vi "spi_full_control.vi"(0 "connection ID":refnum<k5>, 1 "Device":u16(ring) items=["Attenuation", "Clipping", "Enable channel", "Delay line", "ASIC", "Enable L1 ch", "ASIC L1"], 2 "Read/#write":bool, 3 "Data":i32=72, 4 "Register or channel":i32=72, 5 "error out 3":errorcluster, 6 "Read physical":bool, 7 "Id in":i32, 8 "chip delay":i32) -> (9 "Data to send hex":string, 11 "Data to send dec":u32, 13 "hex integer string":string, 14 "connection ID out":refnum<k5>, 15 "Id out":i32=72, 16 "data out serial":string, 17 "data read value":u32, 19 "error out 2":errorcluster)   [LabVIEW 2012]
panel:
  out "Data out 2":string
  out "Data out":string
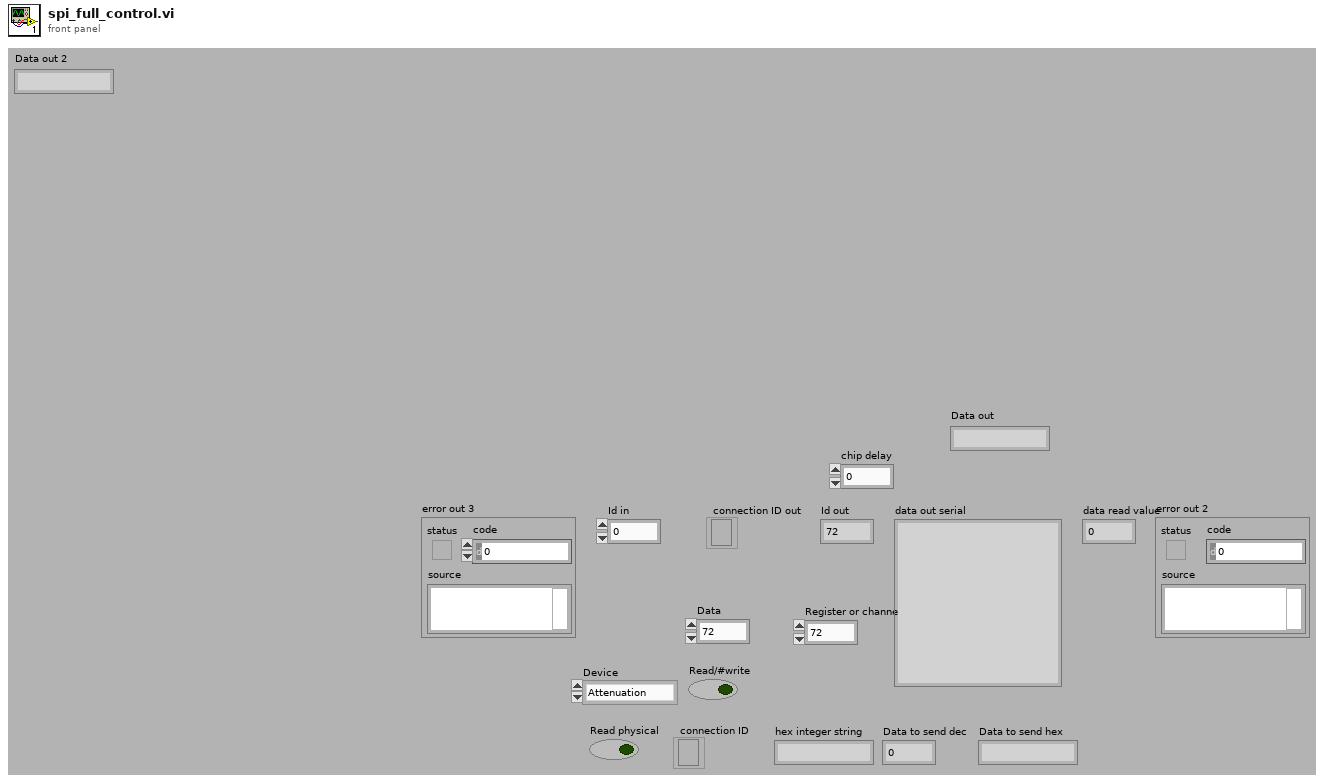
[diagram p1: front panel]
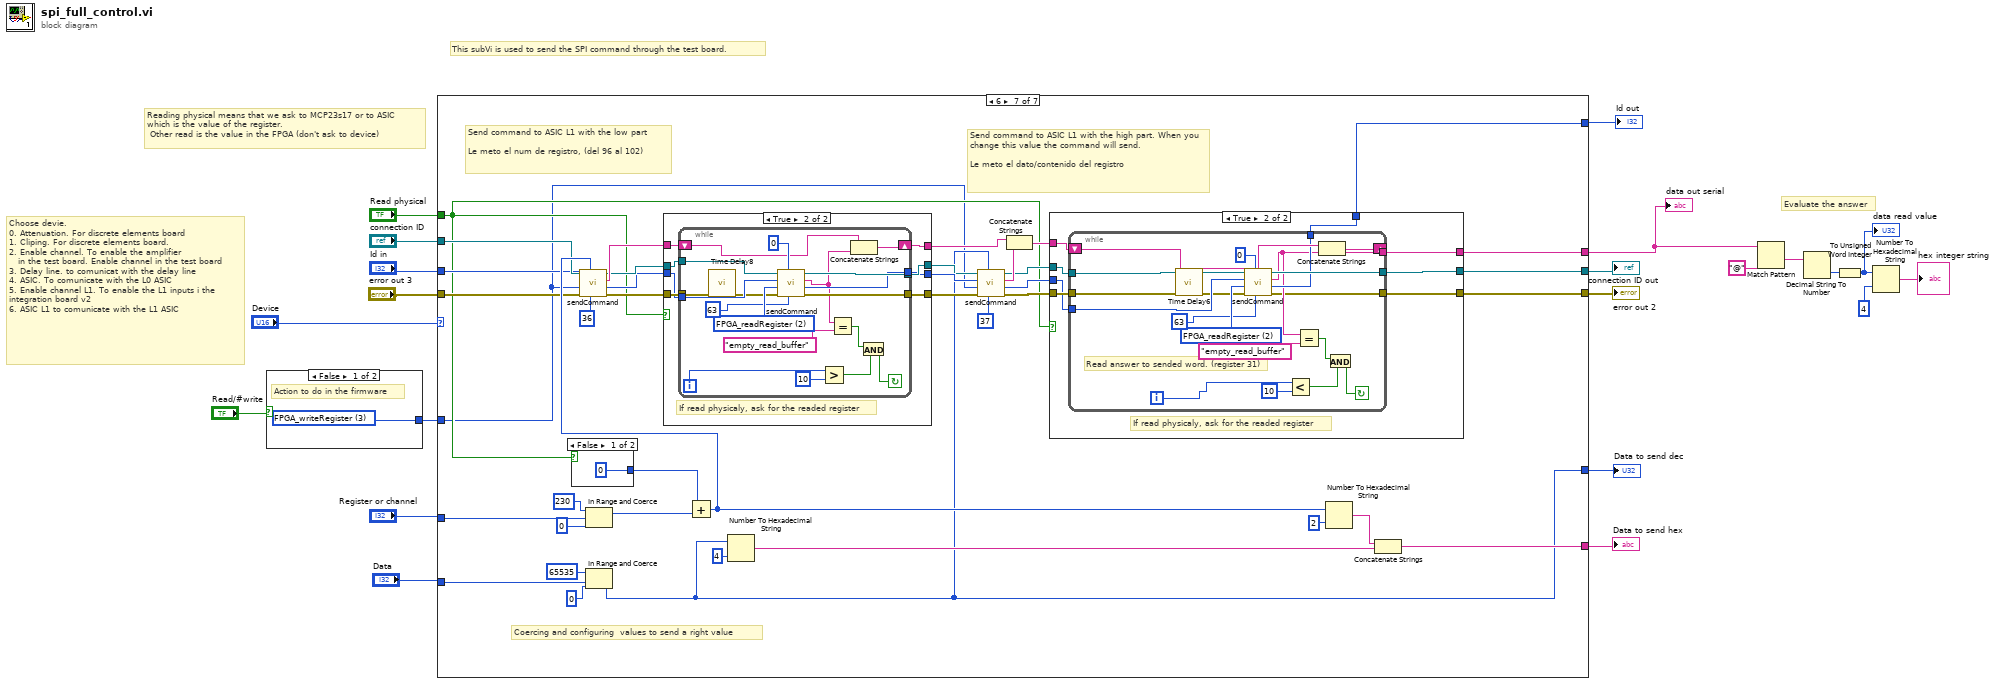
[diagram p0: block diagram]
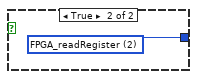
[diagram p2: hidden frame]
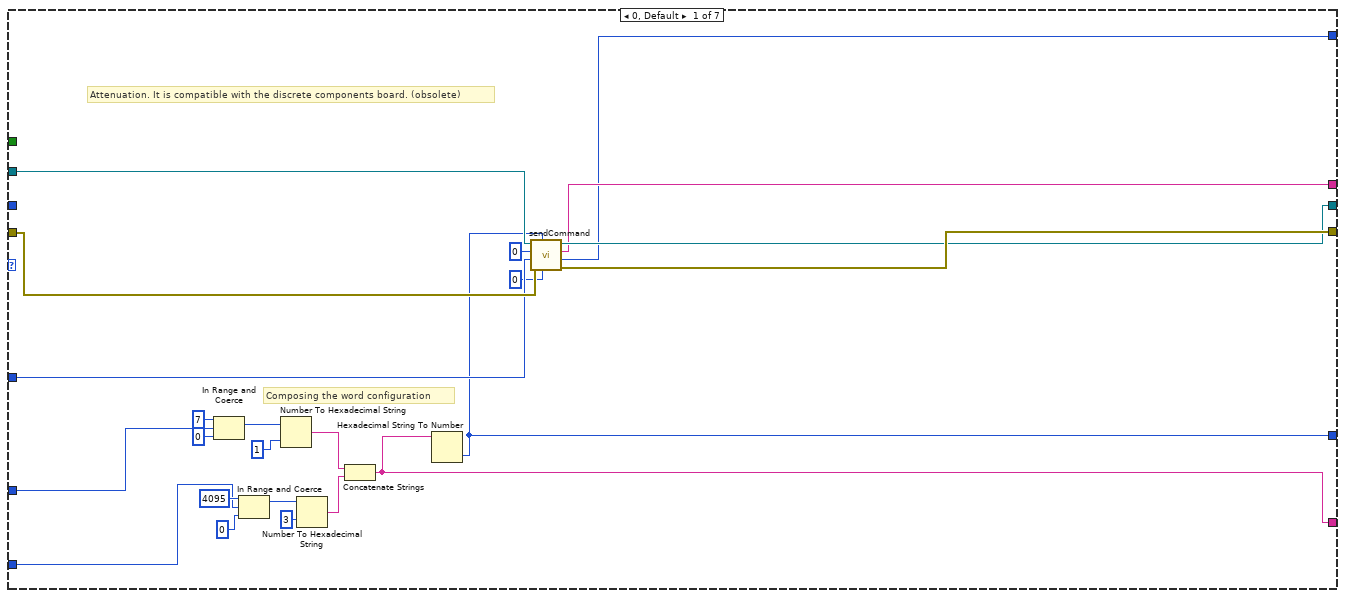
[diagram p3: hidden frame]
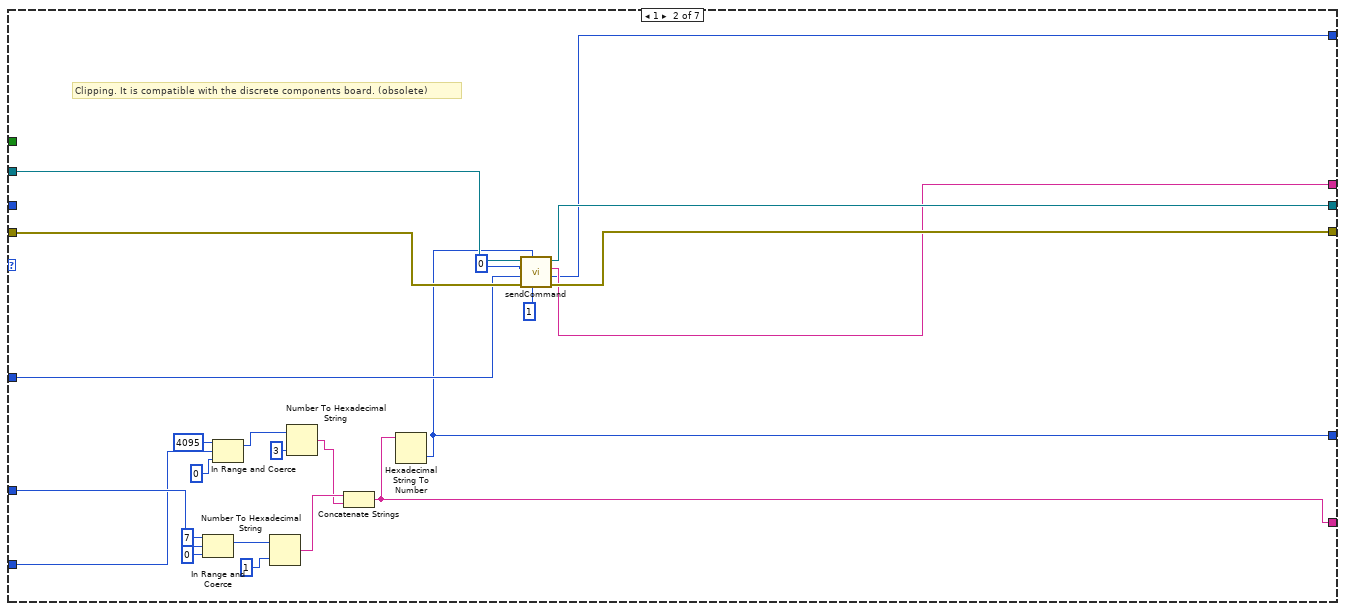
[diagram p4: hidden frame]
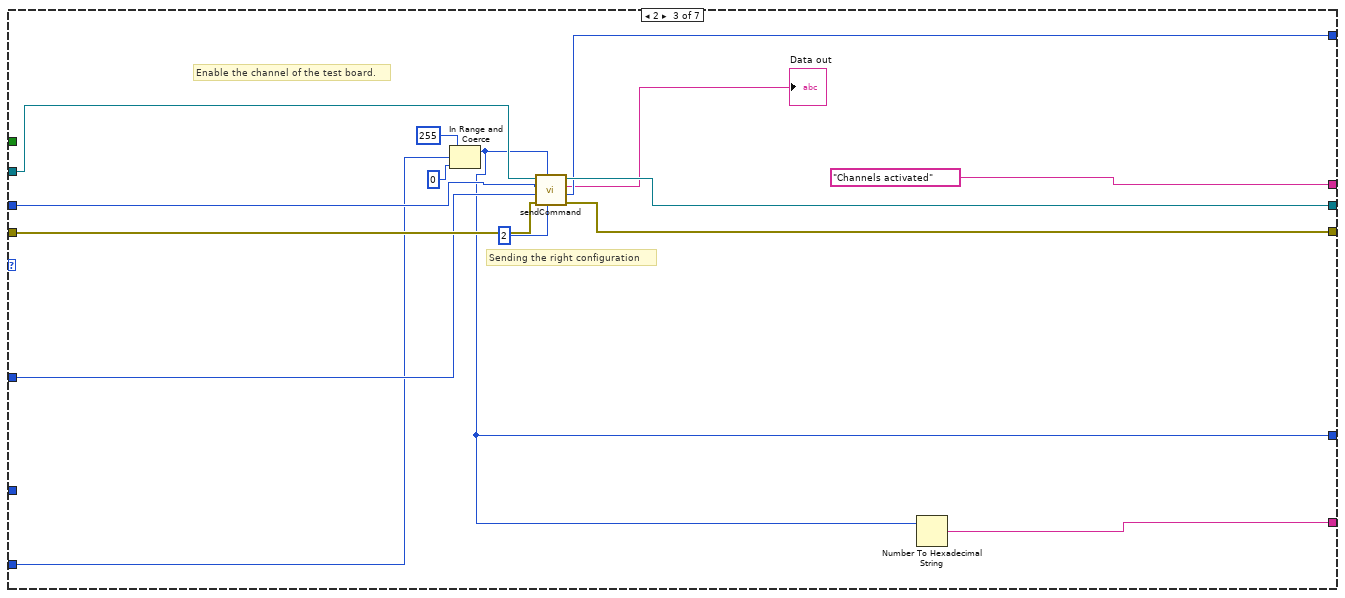
[diagram p5: hidden frame]
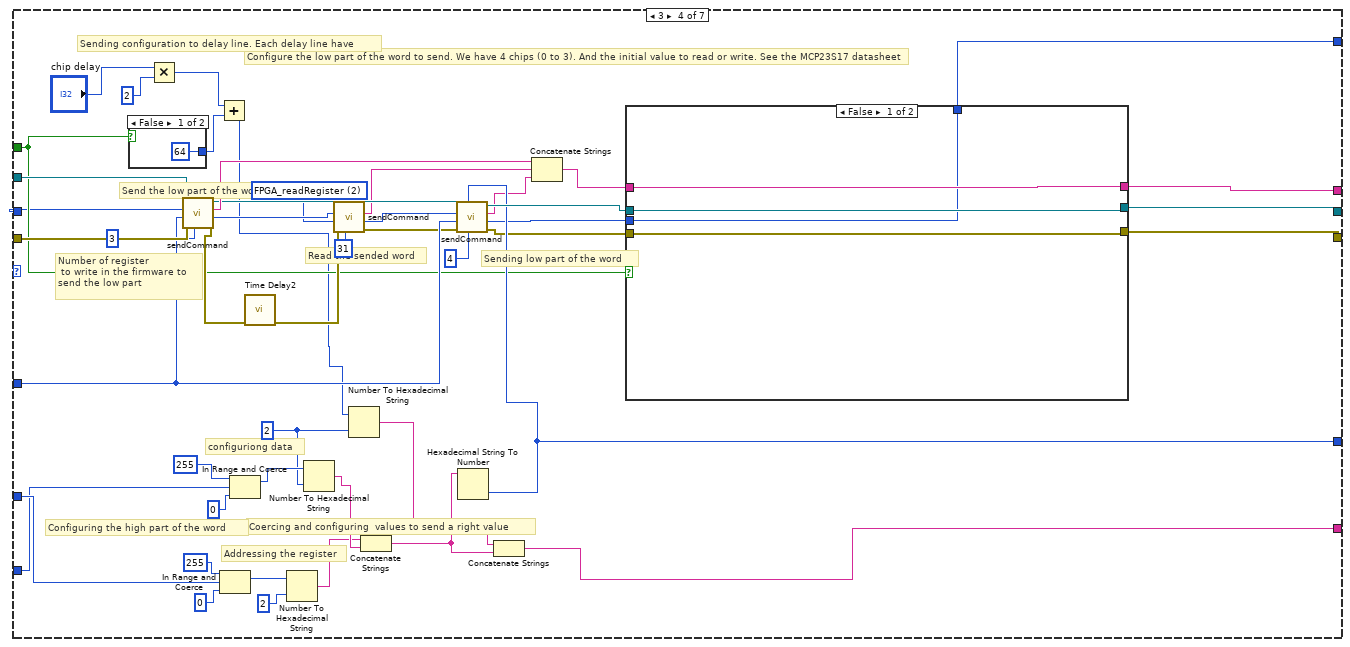
[diagram p6: hidden frame]
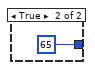
[diagram p7: hidden frame]
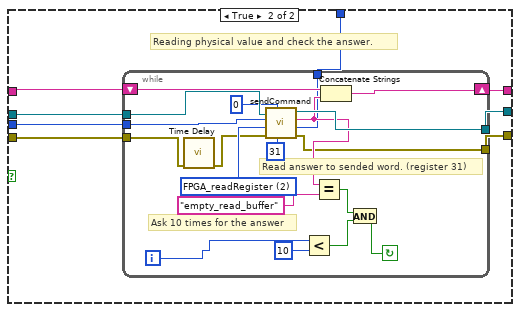
[diagram p8: hidden frame]
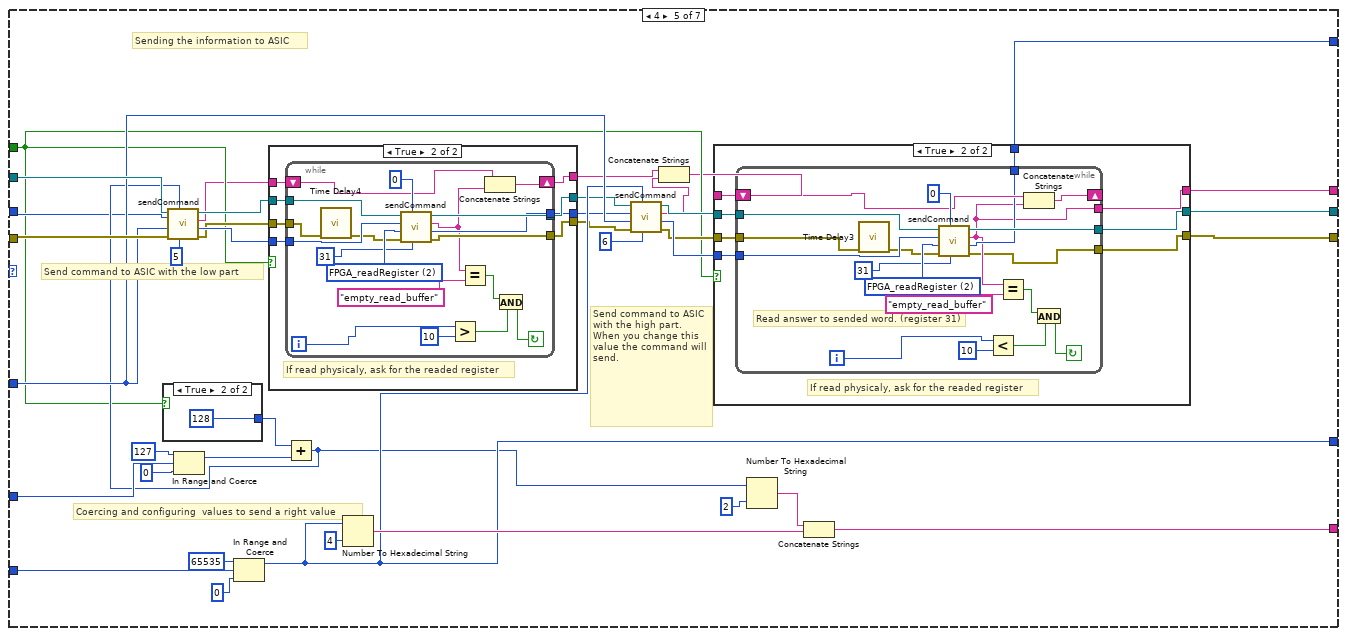
[diagram p9: hidden frame]
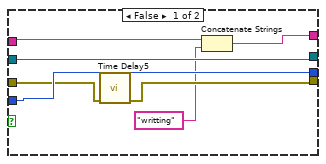
[diagram p10: hidden frame]
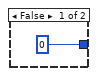
[diagram p11: hidden frame]
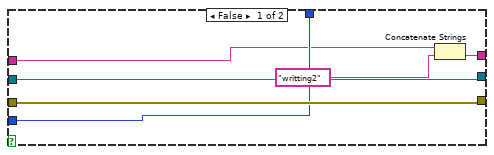
[diagram p12: hidden frame]
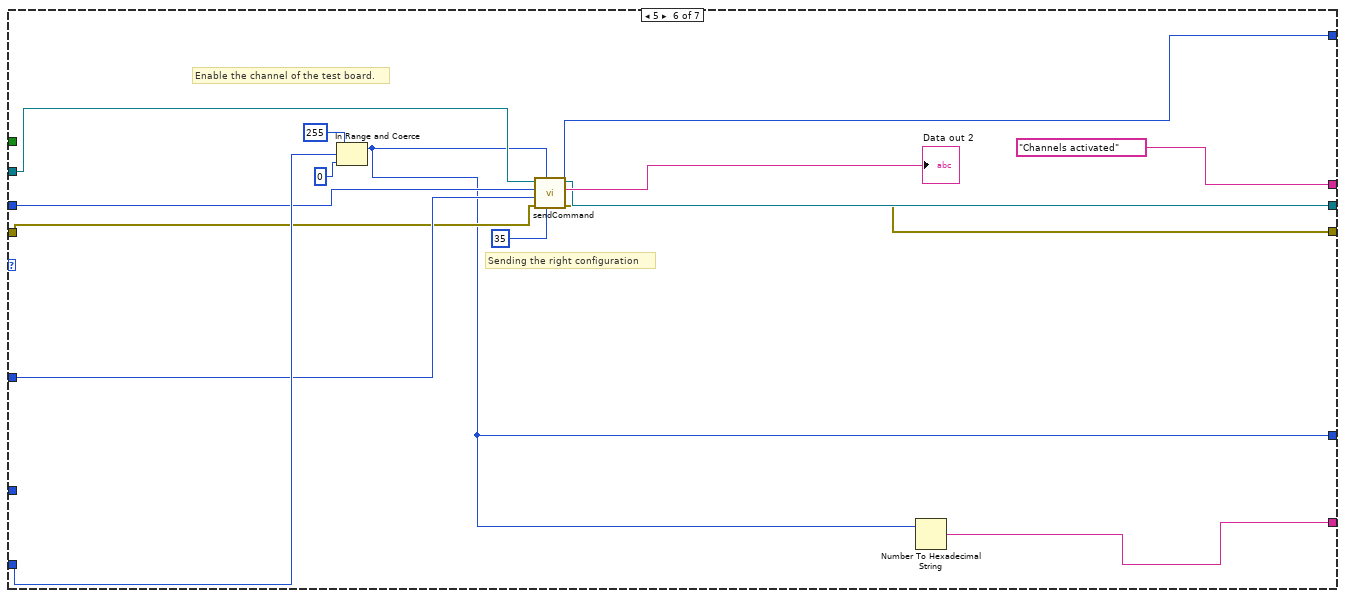
[diagram p13: hidden frame]
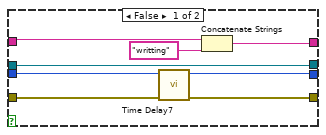
[diagram p14: hidden frame]
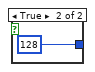
[diagram p15: hidden frame]
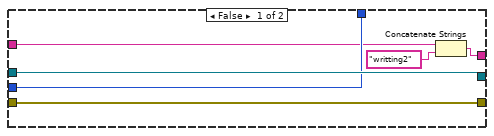
[diagram p16: hidden frame]
diagram:
  # "Reading physical means that we ask to MCP23s17 or to ASIC \nwhich is the value of the register.\n Other read is the value in the FPGA (don't ask to device)"
  # "Evaluate the answer"
  # "Choose devie.\n0. Attenuation. For discrete elements board\n1. Cliping. For discrete elements board.\n2. Enable channel. To enable the amplifier \n   in the test board. Enable channel in the test board\n3. Delay line. to comunicat with the delay line\n4. ASIC. To comunicate with the L0 ASIC\n5. Enable channel L1. To enable the L1 inputs i the integration board v2\n6. ASIC L1 to comunicate with the L1 ASIC"
  # "This subVi is used to send the SPI command through the test board."
  n1 = case shown="False" "Read/#write" {
    tunnel: [w22 w23] -> w9
    frame False {
      w22 = u16 3 items=["sendCommand"=9, "FPGA_writeRegister"=3, "FPGA_readRegister"=2, "uC_writeRegister"=1, "uC_readRegister"=0] ("Action")
      # "Action to do in the firmware"
    }
    frame True {
      w23 = u16 2 items=["sendCommand"=9, "FPGA_writeRegister"=3, "FPGA_readRegister"=2, "uC_writeRegister"=1, "uC_readRegister"=0] ("Action")
    }
  }
  n2 = case shown="6" "Device" {
    tunnel: [w44 w67 w80 w106 w179 w276 w298] -> w7
    tunnel: "error out 3" -> [w45 w69 w83 w132 w192 w282 w292]
    tunnel: "connection ID" -> [w46 w68 w82 w131 w193 w280 w294]
    tunnel: [w43 w66 w81 w105 w187 w277 w297] -> w6
    tunnel: w9 -> [w31 w63 w79 w130 w191 w283 w289]
    tunnel: "Register or channel" -> [w26 w62 _ w118 w189 _ w301]
    tunnel: "Data" -> [w27 w57 w75 w117 w190 w284 w300]
    tunnel: [w25 w48 "Channels activated" ("data out") w104 w180 "Channels activated" ("data out") w296] -> w18
    tunnel: [w29 w50 w74 w116 w184 w279 w291] -> w13
    tunnel: [w28 w49 w72 w111 w188 w278 w299] -> w14
    tunnel: "Read physical" -> [_ _ _ w91 w172 _ w290]
    tunnel: "Id in" -> [_ _ w78 w85 w182 w281 w293]
    tunnel: [w24 w47 w71 w92 w170 w274 w295] -> w3
    frame 0, Default {
      # "Attenuation. It is compatible with the discrete components board. (obsolete)"
      # "Composing the word configuration"
      n3 = In Range and Coerce(upper limit=7, x=w26, lower limit=0) -> (coerced(x)=w41:i32)  [unwired: 1 out]
      n4 = In Range and Coerce(upper limit=4095, x=w27, lower limit=0) -> (coerced(x)=w37:i32)  [unwired: 1 out]
      n5 = Number To Hexadecimal String(1:i16 1 ("width (-)"), 2:w41) -> (0:w34:string)
      n6 = Number To Hexadecimal String(1:i16 3 ("width (-)"), 2:w37) -> (0:w33:string)
      n7 = Concatenate Strings(w34, w33) -> (w28:string)
      n8 = Hexadecimal String To Number(string=w28) -> (number=w29:u32)  [unwired: 2 in, 1 out]
      n9 = call "sendCommand.vi"("Address"=0, "Data"=w29, "error in"=w45, "Action"=w31, "id_in"=0, "connection ID"=w46) -> ("error out"=w44:errorcluster, "id_out"=w24:i32, "Data out"=w25:string, "connection ID out"=w43:refnum<k5>)  [unwired: 1 in, 1 out]
    }
    frame 1 {
      # "Clipping. It is compatible with the discrete components board. (obsolete)"
      n10 = In Range and Coerce(upper limit=7, x=w62, lower limit=0) -> (coerced(x)=w61:i32)  [unwired: 1 out]
      n11 = In Range and Coerce(upper limit=4095, x=w57, lower limit=0) -> (coerced(x)=w56:i32)  [unwired: 1 out]
      n12 = Number To Hexadecimal String(1:i16 1 ("width (-)"), 2:w61) -> (0:w53:string)
      n13 = Number To Hexadecimal String(1:i16 3 ("width (-)"), 2:w56) -> (0:w52:string)
      n14 = Concatenate Strings(w53, w52) -> (w49:string)
      n15 = Hexadecimal String To Number(string=w49) -> (number=w50:u32)  [unwired: 2 in, 1 out]
      n16 = call "sendCommand.vi"("Address"=1, "Data"=w50, "error in"=w69, "Action"=w63, "id_in"=0 ("id"), "connection ID"=w68) -> ("error out"=w67:errorcluster, "id_out"=w47:i32, "Data out"=w48:string, "connection ID out"=w66:refnum<k5>)  [unwired: 1 in, 1 out]
    }
    frame 2 {
      # "Sending the right configuration"
      # "Enable the channel of the test board."
      n17 = In Range and Coerce(upper limit=255, x=w75, lower limit=0) -> (coerced(x)=w74:i32)  [unwired: 1 out]
      n18 = call "sendCommand.vi"("Address"=2, "Data"=w74, "error in"=w83, "Action"=w79, "id_in"=w78, "connection ID"=w82) -> ("error out"=w80:errorcluster, "id_out"=w71:i32, "Data out"=→"Data out":string, "connection ID out"=w81:refnum<k5>)  [unwired: 1 in, 1 out]
      n19 = Number To Hexadecimal String(2:w74) -> (0:w72:string)  [unwired: 1 in]
    }
    frame 3 {
      w97 = u16 2 items=["sendCommand"=9, "FPGA_writeRegister"=3, "FPGA_readRegister"=2, "uC_writeRegister"=1, "uC_readRegister"=0] ("Action")
      w114 = i16 2 ("width (-)")
      # "Coercing and configuring  values to send a right value"
      # "Number of register\n to write in the firmware to \nsend the low part"
      # "Sending low part of the word"
      # "configuriong data"
      # "Addressing the register"
      # "Configuring the high part of the word"
      # "Read the sended word"
      # "Send the low part of the word"
      # "Configure the low part of the word to send. We have 4 chips (0 to 3). And the initial value to read or write. See the MCP23S17 datasheet"
      # "Sending configuration to delay line. Each delay line have"
      n20 = case shown="False" w91 {
        tunnel: [64 ("Address") 65 ("Address")] -> w88
        frame False {
        }
        frame True {
        }
      }
      n21 = Multiply(x="chip delay", y=2) -> (x*y=w89:i32)
      n22 = Add(x=w89, y=w88) -> (x+y=w87:i32)
      n23 = call "sendCommand.vi"("Address"=3, "Data"=w87, "error in"=w132, "Action"=w130, "id_in"=w85, "connection ID"=w131) -> ("error out"=w93:errorcluster, "id_out"=w100:i32, "Data out"=w110:string, "connection ID out"=w102:refnum<k5>)  [unwired: 1 in, 1 out]
      n24 = In Range and Coerce(upper limit=255, x=w118, lower limit=0) -> (coerced(x)=w126:i32)  [unwired: 1 out]
      n25 = In Range and Coerce(upper limit=255, x=w117, lower limit=0) -> (coerced(x)=w122:i32)  [unwired: 1 out]
      n26 = call "Time Delay2"("error in (no error)"=w93) -> ("error out"=w94:errorcluster)  [unwired: 10 in]
      n27 = Number To Hexadecimal String(1:i16 2 ("width (-)"), 2:w126) -> (0:w115:string)
      n28 = Number To Hexadecimal String(1:w114, 2:w122) -> (0:w119:string)
      n29 = call "sendCommand.vi"("Address"=31, "error in"=w94, "Action"=w97, "id_in"=w100, "connection ID"=w102) -> ("error out"=w103:errorcluster, "id_out"=w99:i32, "Data out"=w98:string, "connection ID out"=w101:refnum<k5>)  [unwired: 2 in, 1 out]
      n30 = Number To Hexadecimal String(1:w114, 2:w87) -> (0:w113:string)
      n31 = Concatenate Strings(w115, w119) -> (w112:string)
      n32 = Hexadecimal String To Number(string=w112) -> (number=w116:u32)  [unwired: 2 in, 1 out]
      n33 = call "sendCommand.vi"("Address"=4, "Data"=w116, "error in"=w103, "Action"=w130, "id_in"=w99, "connection ID"=w101) -> ("error out"=w95:errorcluster, "id_out"=w107:i32, "Data out"=w109:string, "connection ID out"=w127:refnum<k5>)  [unwired: 1 in, 1 out]
      n34 = Concatenate Strings(w113, w112) -> (w111:string)
      n35 = Concatenate Strings(w110, w98, w109) -> (w108:string)
      n36 = case shown="False" w91 {
        tunnel: w127 -> [w137 w146]
        tunnel: w95 -> [w138 w145]
        tunnel: [w138 w142] -> w106
        tunnel: [w137 w143] -> w105
        tunnel: [w136 w144] -> w104
        tunnel: w108 -> [w136 w141]
        tunnel: w107 -> [w135 w140]
        tunnel: [w135 w139] -> w92
        frame False {
        }
        frame True {
          # "Reading physical value and check the answer."
          n37 = while {
            tunnel: w145 -> [w149]
            tunnel: [w150] -> w142
            tunnel: [w155] -> w143
            tunnel: w146 -> [w159]
            shift-right: [w152] -> w144
            shift-left: w141 -> [w154]
            tunnel: w140 -> [w151]
            tunnel: [w147] -> w139
            i -> [w160]
            stop <- w161 continue-if-true
            w158 = u16 2 items=["sendCommand"=9, "FPGA_writeRegister"=3, "FPGA_readRegister"=2, "uC_writeRegister"=1, "uC_readRegister"=0] ("Action 2")
            # "Read answer to sended word. (register 31)"
            # "Ask 10 times for the answer"
            n38 = call "Time Delay"("error in (no error)"=w149) -> ("error out"=w148:errorcluster)  [unwired: 10 in]
            n39 = call "sendCommand.vi"("Address"=31, "Data"=0, "error in"=w148, "Action"=w158, "id_in"=w151, "connection ID"=w159) -> ("error out"=w150:errorcluster, "id_out"=w147:i32, "Data out"=w153:string, "connection ID out"=w155:refnum<k5>)  [unwired: 1 in, 1 out]
            n40 = Less?(x=w160, y=10) -> (x < y?=w163:bool)
            n41 = Equal?(x=w153, y="empty_read_buffer") -> (x = y?=w164:bool)
            n42 = Concatenate Strings(w154, w153) -> (w152:string)
            n43 = And(x=w164, y=w163) -> (x .and. y?=w161:bool)
          }
        }
      }
    }
    frame 4 {
      # "Coercing and configuring  values to send a right value"
      # "Send command to ASIC with the high part. When you change this value the command will send."
      # "Send command to ASIC with the low part"
      # "Sending the information to ASIC"
      n44 = case shown="True" w172 {
        tunnel: [0 ("Address") 128 ("Address")] -> w186
        frame False {
        }
        frame True {
        }
      }
      n45 = In Range and Coerce(upper limit=127, x=w189, lower limit=0) -> (coerced(x)=w185:i32)  [unwired: 1 out]
      n46 = In Range and Coerce(upper limit=65535, x=w190, lower limit=0) -> (coerced(x)=w184:i32)  [unwired: 1 out]
      n47 = Add(x=w186, y=w185) -> (x+y=w183:i32)
      n48 = call "sendCommand.vi"("Address"=5, "Data"=w183, "error in"=w192, "Action"=w191, "id_in"=w182, "connection ID"=w193) -> ("error out"=w173:errorcluster, "id_out"=w175:i32, "Data out"=w166:string, "connection ID out"=w174:refnum<k5>)  [unwired: 1 in, 1 out]
      n49 = case shown="True" w172 {
        tunnel: w174 -> [w211 w219]
        tunnel: w173 -> [w209 w218]
        tunnel: [w208 w217] -> w177
        tunnel: [w211 w216] -> w176
        tunnel: [w206 w214] -> w169
        tunnel: w175 -> [w210 w215]
        tunnel: [w210 w213] -> w171
        tunnel: w166 -> [w205 w212]
        frame False {
          n50 = call "Time Delay5"("error in (no error)"=w209) -> ("error out"=w208:errorcluster)  [unwired: 10 in]
          n51 = Concatenate Strings(w205, "writting" ("Data out")) -> (w206:string)
        }
        frame True {
          # "If read physicaly, ask for the readed register"
          n52 = while {
            tunnel: w218 -> [w226]
            tunnel: [w224] -> w217
            tunnel: [w232] -> w216
            tunnel: w219 -> [w228]
            tunnel: w215 -> [w231]
            tunnel: [w223] -> w213
            shift-right: [w220] -> w214
            shift-left: w212 -> [w222]
            i -> [w233]
            stop <- w234 continue-if-true
            w230 = u16 2 items=["sendCommand"=9, "FPGA_writeRegister"=3, "FPGA_readRegister"=2, "uC_writeRegister"=1, "uC_readRegister"=0] ("Action 2")
            n53 = call "Time Delay4"("error in (no error)"=w226) -> ("error out"=w225:errorcluster)  [unwired: 10 in]
            n54 = call "sendCommand.vi"("Address"=31, "Data"=0, "error in"=w225, "Action"=w230, "id_in"=w231, "connection ID"=w228) -> ("error out"=w224:errorcluster, "id_out"=w223:i32, "Data out"=w221:string, "connection ID out"=w232:refnum<k5>)  [unwired: 1 in, 1 out]
            n55 = Greater?(x=w233, y=10) -> (0:w236:bool)
            n56 = Equal?(x=w221, y="empty_read_buffer") -> (x = y?=w237:bool)
            n57 = Concatenate Strings(w222, w221) -> (w220:string)
            n58 = And(x=w237, y=w236) -> (x .and. y?=w234:bool)
          }
        }
      }
      n59 = Number To Hexadecimal String(1:i16 4 ("width (-)"), 2:w184) -> (0:w194:string)
      n60 = call "sendCommand.vi"("Address"=6, "Data"=w184, "error in"=w177, "Action"=w191, "id_in"=w171, "connection ID"=w176) -> ("error out"=w178:errorcluster, "id_out"=w181:i32, "Data out"=w168:string, "connection ID out"=w202:refnum<k5>)  [unwired: 1 in, 1 out]
      n61 = Concatenate Strings(w169, w168) -> (w167:string)
      n62 = case shown="True" w172 {
        tunnel: w202 -> [w245 w254]
        tunnel: w178 -> [w246 w253]
        tunnel: [w246 w252] -> w179
        tunnel: [w245 w251] -> w187
        tunnel: [w243 w247] -> w180
        tunnel: w181 -> [w244 w250]
        tunnel: w167 -> [w241 w249]
        tunnel: [w244 w248] -> w170
        frame False {
          n63 = Concatenate Strings(w241, "writting2" ("Data out")) -> (w243:string)
        }
        frame True {
          # "If read physicaly, ask for the readed register"
          n64 = while {
            tunnel: w253 -> [w261]
            tunnel: [w255] -> w252
            tunnel: [w267] -> w251
            tunnel: w254 -> [w263]
            tunnel: w250 -> [w266]
            tunnel: [w257] -> w248
            shift-right: [w259] -> _
            shift-left: w249 -> [w258]
            tunnel: [w256] -> w247
            i -> [w268]
            stop <- w269 continue-if-true
            w265 = u16 2 items=["sendCommand"=9, "FPGA_writeRegister"=3, "FPGA_readRegister"=2, "uC_writeRegister"=1, "uC_readRegister"=0] ("Action 2")
            # "Read answer to sended word. (register 31)"
            n65 = call "Time Delay3"("error in (no error)"=w261) -> ("error out"=w260:errorcluster)  [unwired: 10 in]
            n66 = call "sendCommand.vi"("Address"=31, "Data"=0, "error in"=w260, "Action"=w265, "id_in"=w266, "connection ID"=w263) -> ("error out"=w255:errorcluster, "id_out"=w257:i32, "Data out"=w256:string, "connection ID out"=w267:refnum<k5>)  [unwired: 1 in, 1 out]
            n67 = Less?(x=w268, y=10) -> (x < y?=w271:bool)
            n68 = Equal?(x=w256, y="empty_read_buffer") -> (x = y?=w272:bool)
            n69 = Concatenate Strings(w258, w256) -> (w259:string)
            n70 = And(x=w272, y=w271) -> (x .and. y?=w269:bool)
          }
        }
      }
      n71 = Number To Hexadecimal String(1:i16 2 ("width (-)"), 2:w183) -> (0:w195:string)
      n72 = Concatenate Strings(w195, w194) -> (w188:string)
    }
    frame 5 {
      # "Sending the right configuration"
      # "Enable the channel of the test board."
      n73 = In Range and Coerce(upper limit=255, x=w284, lower limit=0) -> (coerced(x)=w279:i32)  [unwired: 1 out]
      n74 = call "sendCommand.vi"("Address"=35, "Data"=w279, "error in"=w282, "Action"=w283, "id_in"=w281, "connection ID"=w280) -> ("error out"=w276:errorcluster, "id_out"=w274:i32, "Data out"=→"Data out 2":string, "connection ID out"=w277:refnum<k5>)  [unwired: 1 in, 1 out]
      n75 = Number To Hexadecimal String(2:w279) -> (0:w278:string)  [unwired: 1 in]
    }
    frame 6 {
      # "Coercing and configuring  values to send a right value"
      # "Send command to ASIC L1 with the high part. When you change this value the command will send.\n\nLe meto el dato/contenido del registro"
      # "Send command to ASIC L1 with the low part\n\nLe meto el num de registro, (del 96 al 102)"
      n76 = case shown="False" w290 {
        tunnel: [0 ("Address") 128 ("Address")] -> w313
        frame False {
        }
        frame True {
        }
      }
      n77 = In Range and Coerce(upper limit=230, x=w301, lower limit=0) -> (coerced(x)=w314:i32)  [unwired: 1 out]
      n78 = In Range and Coerce(upper limit=65535, x=w300, lower limit=0) -> (coerced(x)=w291:i32)  [unwired: 1 out]
      n79 = Add(x=w313, y=w314) -> (x+y=w315:i32)
      n80 = call "sendCommand.vi"("Address"=36, "Data"=w315, "error in"=w292, "Action"=w289, "id_in"=w293, "connection ID"=w294) -> ("error out"=w322:errorcluster, "id_out"=w320:i32, "Data out"=w327:string, "connection ID out"=w321:refnum<k5>)  [unwired: 1 in, 1 out]
      n81 = case shown="True" w290 {
        tunnel: w321 -> [w334 w342]
        tunnel: w322 -> [w332 w341]
        tunnel: [w331 w340] -> w318
        tunnel: [w334 w339] -> w319
        tunnel: [w329 w337] -> w324
        tunnel: w320 -> [w333 w338]
        tunnel: [w333 w336] -> w323
        tunnel: w327 -> [w328 w335]
        frame False {
          n82 = call "Time Delay7"("error in (no error)"=w332) -> ("error out"=w331:errorcluster)  [unwired: 10 in]
          n83 = Concatenate Strings(w328, "writting" ("Data out")) -> (w329:string)
        }
        frame True {
          # "If read physicaly, ask for the readed register"
          n84 = while {
            tunnel: w341 -> [w349]
            tunnel: [w347] -> w340
            tunnel: [w355] -> w339
            tunnel: w342 -> [w351]
            tunnel: w338 -> [w354]
            tunnel: [w346] -> w336
            shift-right: [w343] -> w337
            shift-left: w335 -> [w345]
            i -> [w356]
            stop <- w357 continue-if-true
            w353 = u16 2 items=["sendCommand"=9, "FPGA_writeRegister"=3, "FPGA_readRegister"=2, "uC_writeRegister"=1, "uC_readRegister"=0] ("Action 2")
            n85 = call "Time Delay8"("error in (no error)"=w349) -> ("error out"=w348:errorcluster)  [unwired: 10 in]
            n86 = call "sendCommand.vi"("Address"=63, "Data"=0, "error in"=w348, "Action"=w353, "id_in"=w354, "connection ID"=w351) -> ("error out"=w347:errorcluster, "id_out"=w346:i32, "Data out"=w344:string, "connection ID out"=w355:refnum<k5>)  [unwired: 1 in, 1 out]
            n87 = Greater?(x=w356, y=10) -> (0:w359:bool)
            n88 = Equal?(x=w344, y="empty_read_buffer") -> (x = y?=w360:bool)
            n89 = Concatenate Strings(w345, w344) -> (w343:string)
            n90 = And(x=w360, y=w359) -> (x .and. y?=w357:bool)
          }
        }
      }
      n91 = Number To Hexadecimal String(1:i16 4 ("width (-)"), 2:w291) -> (0:w312:string)
      n92 = call "sendCommand.vi"("Address"=37, "Data"=w291, "error in"=w318, "Action"=w289, "id_in"=w323, "connection ID"=w319) -> ("error out"=w317:errorcluster, "id_out"=w316:i32, "Data out"=w325:string, "connection ID out"=w304:refnum<k5>)  [unwired: 1 in, 1 out]
      n93 = Concatenate Strings(w324, w325) -> (w326:string)
      n94 = case shown="True" w290 {
        tunnel: w304 -> [w368 w377]
        tunnel: w317 -> [w369 w376]
        tunnel: [w369 w375] -> w298
        tunnel: [w368 w374] -> w297
        tunnel: [w366 w370] -> w296
        tunnel: w316 -> [w367 w373]
        tunnel: w326 -> [w364 w372]
        tunnel: [w367 w371] -> w295
        frame False {
          n95 = Concatenate Strings(w364, "writting2" ("Data out")) -> (w366:string)
        }
        frame True {
          # "If read physicaly, ask for the readed register"
          n96 = while {
            tunnel: w376 -> [w384]
            tunnel: [w378] -> w375
            tunnel: [w390] -> w374
            tunnel: w377 -> [w386]
            tunnel: w373 -> [w389]
            tunnel: [w380] -> w371
            shift-right: [w382] -> _
            shift-left: w372 -> [w381]
            tunnel: [w379] -> w370
            i -> [w391]
            stop <- w392 continue-if-true
            w388 = u16 2 items=["sendCommand"=9, "FPGA_writeRegister"=3, "FPGA_readRegister"=2, "uC_writeRegister"=1, "uC_readRegister"=0] ("Action 2")
            # "Read answer to sended word. (register 31)"
            n97 = call "Time Delay6"("error in (no error)"=w384) -> ("error out"=w383:errorcluster)  [unwired: 10 in]
            n98 = call "sendCommand.vi"("Address"=63, "Data"=0, "error in"=w383, "Action"=w388, "id_in"=w389, "connection ID"=w386) -> ("error out"=w378:errorcluster, "id_out"=w380:i32, "Data out"=w379:string, "connection ID out"=w390:refnum<k5>)  [unwired: 1 in, 1 out]
            n99 = Less?(x=w391, y=10) -> (x < y?=w394:bool)
            n100 = Equal?(x=w379, y="empty_read_buffer") -> (x = y?=w395:bool)
            n101 = Concatenate Strings(w381, w379) -> (w382:string)
            n102 = And(x=w395, y=w394) -> (x .and. y?=w392:bool)
          }
        }
      }
      n103 = Number To Hexadecimal String(1:i16 2 ("width (-)"), 2:w315) -> (0:w311:string)
      n104 = Concatenate Strings(w311, w312) -> (w299:string)
    }
  }
  "data out serial" <- w18
  "Data to send dec" <- w13
  "Data to send hex" <- w14
  "Id out" <- w3
  "error out 2" <- w7
  "connection ID out" <- w6
  n105 = Match Pattern(string=w18, regular expression="@" ("search string/char (-)")) -> (after substring=w16:string)  [unwired: 1 in, 3 out]
  n106 = Decimal String To Number(string=w16) -> (number=w2:i32)  [unwired: 2 in, 1 out]
  n107 = To Unsigned Word Integer(number=w2) -> (unsigned 16bit integer=w1:u16)
  "data read value" <- w1
  n108 = Number To Hexadecimal String(1:i16 4 ("width (-)"), 2:w1) -> (0:→"hex integer string":string)
